vi "Create Generic Log Message.vi"(6 "Level":T1, 7 "Logger Name":string, 8 "error in (no error)":errorcluster, 10 "Message":string, 11 "Call Chain":string[](array[string])) -> (0 "error out":errorcluster)   [LabVIEW 2016, in "Global_logger.lvlib"]
uses:
  Global_logger.lvlib
  Levels.ctl
  Event.ctl
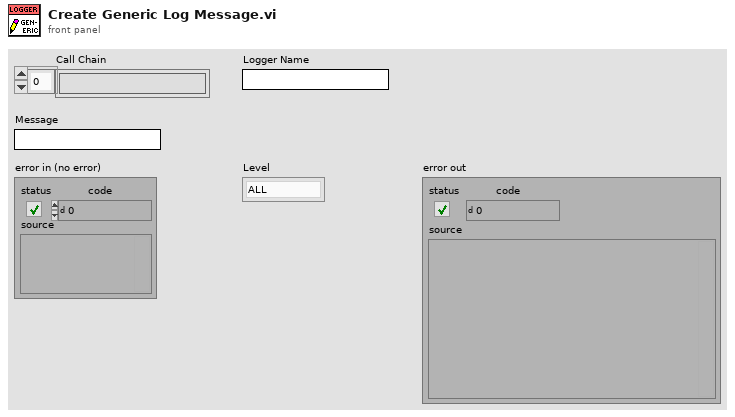
[diagram p1: front panel]
types:
  T1 = typedef "Global_logger.lvlib/Levels.ctl" = enum16{"ALL", "TRACE", "DEBUG", "INFO", "WARN", "ERROR", "FATAL", "OFF"}
  T2 = typedef "Global_logger.lvlib/Event.ctl" = cluster{"Logger Name":string, "Time Stamp":timestamp, "Level":T1, "Source VI":string, "Message":string, "Source App":string}
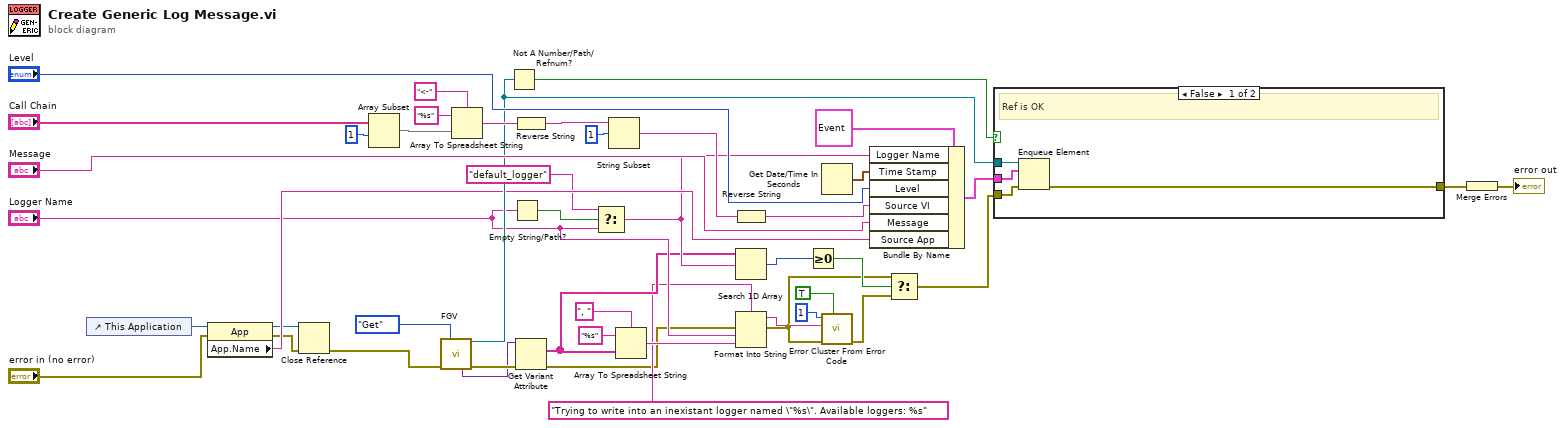
[diagram p0: block diagram]
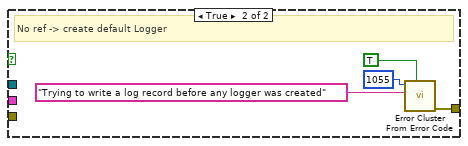
[diagram p2: hidden frame]
diagram:
  n1 = control-ref of="This Application"() -> (w23:refnum<vi>)
  n2 = property class="App"(reference=w23, error in="error in (no error)") -> (reference out=w21:refnum<vi>, error out=w24:errorcluster, "App.Name"=w26:string)
  n3 = Close Reference(reference=w21, error in (no error)=w24) -> (error out=w22:errorcluster)
  n4 = Array Subset(array="Call Chain", index=1) -> (w31:string[])  [unwired: 1 in]
  n5 = call "FGV.vi"("Action"=enum16{"Get", "Set"}."Get", "error in (no error)"=w22) -> ("queue out"=w28:refnum<queue>, "All Named Loggers"=w17:variant, "error out"=w18:errorcluster)  [unwired: 8 in, 3 out]
  n6 = Array To Spreadsheet String(delimiter (Tab)="<-", array=w31, 3:"%s" ("format string")) -> (spreadsheet string=w37:string)
  n7 = Not A Number/Path/Refnum?(number/path/refnum=w28) -> (NaN/Path/Refnum?=w27:bool)
  n8 = Empty String/Path?(string/path="Logger Name") -> (empty?=w20:bool)
  n9 = Reverse String(1:w37) -> (0:w36:string)
  n10 = Get Variant Attribute(Variant=w17, error in=w18) -> (names=w12:string[], error out=w7:errorcluster)  [unwired: 2 in, 2 out]
  n11 = Select(t="default_logger", s=w20, f="Logger Name") -> (s? t:f=w16:string)
  n12 = String Subset(string=w36, offset (0)=1) -> (substring=w34:string)  [unwired: 1 in]
  n13 = Array To Spreadsheet String(delimiter (Tab)=", ", array=w12, 3:"%s" ("format string")) -> (spreadsheet string=w9:string)
  n14 = Reverse String(1:w34) -> (0:w33:string)
  n15 = Search 1D Array(1D array=w12, element=w16) -> (index of element=w15:i32)  [unwired: 1 in]
  n16 = Format Into String(format string="Trying to write into an inexistant logger named \"%s\". Available loggers: %s", error in=w7, "Logger Name", w9) -> (resulting string=w6:string, error out=w2:errorcluster)  [unwired: 1 in]
  n17 = Greater Or Equal To 0?(x=w15) -> (x >= 0?=w4:bool)
  n18 = Get Date/Time In Seconds() -> (seconds since 1Jan1904=w44:timestamp)
  n19 = call <vilib>:"Error Cluster From Error Code.vi"("show call chain? (False)"=TRUE, "error in (no error)"=w2, "error message (\"\")"=w6, "error code (0)"=1) -> ("error out"=w3:errorcluster)  [unwired: 5 in]
  n20 = Bundle By Name(cluster=T2 {"Logger Name"="", "Time Stamp"=timestamp(0 s since 1904-01-01), "Level"=enum."ALL", "Source VI"="", "Message"="", "Source App"=""} ("element"), "Logger Name"=w16, "Time Stamp"=w44, "Level"="Level", "Source VI"=w33, "Message"="Message", "Source App"=w26) -> (w43:T2)
  n21 = Select(t=w2, s=w4, f=w3) -> (s? t:f=w1:errorcluster)
  n22 = case shown="False" w27 {
    tunnel: w43 -> [w50 _]
    tunnel: [w49 w52] -> w30
    tunnel: w28 -> [w48 _]
    tunnel: w1 -> [w47 _]
    frame False {
      # "Ref is OK"
      n23 = Enqueue Element(queue=w48, element=w50, error in (no error)=w47) -> (error out=w49:errorcluster)  [unwired: 1 in, 2 out]
    }
    frame True {
      # "No ref -> create default Logger"
      n24 = call <vilib>:"Error Cluster From Error Code.vi"("show call chain? (False)"=TRUE, "error message (\"\")"="Trying to write a log record before any logger was created" ("error message (\"\")"), "error code (0)"=1055) -> ("error out"=w52:errorcluster)  [unwired: 6 in]
    }
  }
  n25 = Merge Errors(w30) -> (→"error out":errorcluster)
